vi "dfd_FXP Quantizer to Operation.vi"(10 "quantizer":T3={"source"=0, "wl"=16, "iwl"=1, "overflow mode"=enum."Wrap", "rounding mode"=enum."Truncation", "signed?"=TRUE} {"source" items=["Coef a/k"=0, "Coef b/v"=7, "Input"=1, "Output"=2, "Multiplicand"=3, "Product"=4, "Sum"=5, "Delay"=6, "Gain"=8]}) -> (2 "op params":T1={"source"=0, "is floating?"=FALSE, "o-mode"=enum."Wrap", "q-mode"=enum."Nearest", "signed?"=FALSE, "fwl"=0, "high limit"=0.0, "low limit"=0.0, "full range"=0.0} {"source" items=["Coef a/k"=0, "Coef b/v"=7, "Input"=1, "Output"=2, "Multiplicand"=3, "Product"=4, "Sum"=5, "Delay"=6, "Gain"=8]})   [LabVIEW 2017, in "NI_DigFilter_FXP.lvlib"]
uses:
  <vilib>/addons/Digital Filter Design/NI_DigFilter_FXP.lvlib
  <vilib>/addons/Digital Filter Design/_Objects.llb/dfd_Internal Quantization Settings.ctl
  <vilib>/addons/Digital Filter Design/_Objects.llb/dfd_Internal Quantization Srcs.ctl
  <vilib>/addons/Digital Filter Design/_Objects.llb/dfd_FXP Operation.ctl
  <vilib>/addons/Digital Filter Design/NI_DigFilterLicensed.lvlib
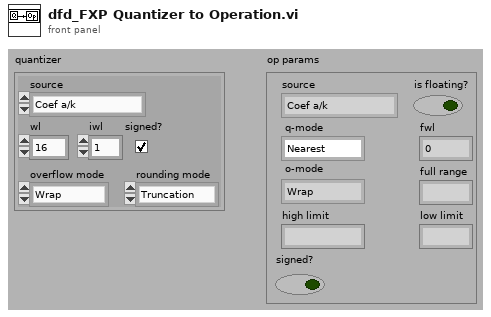
[diagram p1: front panel]
types:
  T1 = typedef "dfd_FXP Operation.ctl" = cluster{"source":T2, "is floating?":bool, "o-mode":enum16{"Saturation", "Wrap"}, "q-mode":enum16{"Nearest", "Truncation"}, "signed?":bool, "fwl":i16, "high limit":ext, "low limit":ext, "full range":ext}
  T2 = typedef "NI_DigFilterLicensed.lvlib/dfd_Internal Quantization Srcs.ctl" = u16
  T3 = typedef "NI_DigFilterLicensed.lvlib/dfd_Internal Quantization Settings.ctl" = cluster{"source":T2, "wl":i16, "iwl":i16, "overflow mode":enum16{"Saturation", "Wrap"}, "rounding mode":enum16{"Nearest", "Truncation"}, "signed?":bool}
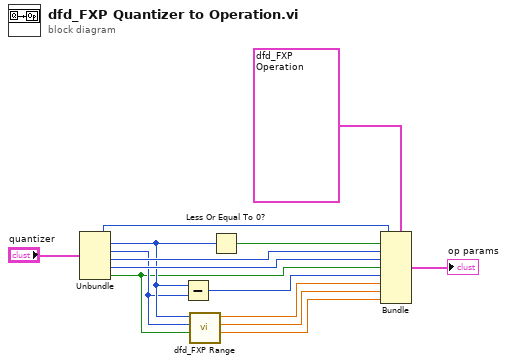
[diagram p0: block diagram]
diagram:
  n1 = Unbundle("quantizer") -> ("source"=w12:T2, "wl"=w6:i16, "iwl"=w5:i16, "overflow mode"=w9:enum16{"Saturation", "Wrap"}, "rounding mode"=w8:enum16{"Nearest", "Truncation"}, "signed?"=w4:bool)
  n2 = Subtract(x=w6, y=w5) -> (x-y=w7:i16)
  n3 = call <vilib>:"dfd_FXP Range.vi"("signed?"=w4, "iwl"=w5, "wl"=w6) -> ("full range"=w1:ext, "low"=w2:ext, "high"=w3:ext)  [unwired: 6 out]
  n4 = Less Or Equal To 0?(x=w6) -> (x <= 0?=w11:bool)
  n5 = Bundle(cluster=T1 {"source"=0, "is floating?"=FALSE, "o-mode"=enum."Saturation", "q-mode"=enum."Nearest", "signed?"=FALSE, "fwl"=0, "high limit"=0.0, "low limit"=0.0, "full range"=0.0} ("op params"), "source"=w12, "is floating?"=w11, "o-mode"=w9, "q-mode"=w8, "signed?"=w4, "fwl"=w7, "high limit"=w3, "low limit"=w2, "full range"=w1) -> (→"op params":T1)
